vi "S4GUI.vi"(7 "Tab ObsEng":enum32{"Obs", "CCD modes", "Eng"}(tab)) -> ()   [LabVIEW 2018] (continued)
                    n784 = property on="Vertical Binning 2" class="DigNum (strict)"("Blinking"=w1441) -> ()  [unwired: 2 in, 2 out]
                    n785 = property on="Horizontal Binning 2" class="DigNum (strict)"("Blinking"=w1443) -> ()  [unwired: 2 in, 2 out]
                    n786 = property on="CCD EM Gain 2" class="DigNum (strict)"("Blinking"=w1438) -> ()  [unwired: 2 in, 2 out]
                    n787 = property on="Shutter Mode 2" class="Ring (strict)"("Blinking"=w1439) -> ()  [unwired: 2 in, 2 out]
                    n788 = property on="Shutter TTL 2" class="Ring (strict)"("Blinking"=w1437) -> ()  [unwired: 2 in, 2 out]
                    n789 = Not(x=w1415) -> (.not. x?=w1430:bool)
                    n790 = Not(x=w1411) -> (.not. x?=w1433:bool)
                    n791 = Not(x=w1410) -> (.not. x?=w1431:bool)
                    n792 = Not(x=w1409) -> (.not. x?=w1432:bool)
                    n793 = Not(x=w1414) -> (.not. x?=w1435:bool)
                    n794 = Not(x=w1413) -> (.not. x?=w1434:bool)
                    n795 = Not(x=w1412) -> (.not. x?=w1436:bool)
                    n796 = property on="Acquisition Mode 2" class="Ring (strict)"("Blinking"=w1430) -> ()  [unwired: 2 in, 2 out]
                    n797 = property on="Readout Rate 2" class="Ring (strict)"("Blinking"=w1433) -> ()  [unwired: 2 in, 2 out]
                    n798 = property on="Vertical Shift Speed 2" class="Ring (strict)"("Blinking"=w1431) -> ()  [unwired: 2 in, 2 out]
                    n799 = property on="CCD EM Mode 2" class="Ring (strict)"("Blinking"=w1432) -> ()  [unwired: 2 in, 2 out]
                    n800 = property on="Trigger Mode 2" class="Ring (strict)"("Blinking"=w1435) -> ()  [unwired: 2 in, 2 out]
                    n801 = property on="Read Mode 2" class="Ring (strict)"("Blinking"=w1434) -> ()  [unwired: 2 in, 2 out]
                    n802 = property on="Pre-amplification Gain 2" class="Ring (strict)"("Blinking"=w1436) -> ()  [unwired: 2 in, 2 out]
                  }
                }
                n803 = local read "Cameras Cluster"() -> (w1400:T7)
                n804 = Bundle By Name(cluster=w1400, "Current Configuration.Image Initial Line 2"=w1363, "Current Configuration.Image Initial Column 2"=w1361, "Current Configuration.Image Final Line 2"=w1364, "Current Configuration.Image FInal Column 2"=w1362, "Current Configuration.Vertical Binning 2"=w1367, "Current Configuration.Horizontal Binning 2"=w1398, "Current Configuration.Pre-amplification Gain 2"=w1366, "Current Configuration.CCD EM Gain 2"=w1365, "Current Configuration.Readout Rate 2"=w1360, "Current Configuration.Shutter Openning Time 2"=w1397, "Current Configuration.Shutter Closing Time 2"=w1396, "Current Configuration.Vertical Shift Speed 2"=w1395, "Current Configuration.Read Mode 2"=w1394, "Current Configuration.Vertical Clock Voltage 2"=w1393, "Current Configuration.A/D Channel 2"=w1392, "Current Configuration.Shutter Mode 2"=w1389, "Current Configuration.Shutter TTL 2"=w1390, "Current Configuration.Trigger Mode 2"=w1368, "Current Configuration.Frame Transfer 2"=w1369, "Current Configuration.Acquisition Mode 2"=w1391, "Current Configuration.CCD EM Mode 2"=w1359) -> (w1399:T7)
                n805 = local write "PA2"(w1354) -> ()
                n806 = local write "B2"(w1353) -> ()
                n807 = local write "EA2"(w1355) -> ()
                n808 = local write "SI2"(w1350) -> ()
                n809 = local write "RO2"(w1351) -> ()
                n810 = local write "G2"(w1352) -> ()
                n811 = local write "Cameras Cluster"(w1399) -> ()
                n812 = Compound Arithmetic op=AND(w1374, w1373, w1372, w1371, w1347, w1346, w1370, w1381, w1380, w1379, w1378, w1377, w1376, w1375, w1388, w1387, w1386, w1385, w1384, w1383, w1382) -> (w1345:bool)
                "CCD checked 2" <- w1345
                n813 = disable-structure shown="Disabled" {
                  disable-tunnel: w1345 -> [w1402 _]
                  frame Disabled {
                    n814 = Select(t=u32 1244955, s=w1402, f=u32 16718848) -> (s? t:f=w1405:u32)
                    n815 = property on="CCD checked 2" class="Bool (strict)"("Caption.BG Color"=w1405) -> ()  [unwired: 2 in, 2 out]
                  }
                  frame Enabled {
                  }
                }
                n816 = property on="Acquisition Mode 2" class="Ring (strict)"("DisabledEnum"=w1348) -> ()  [unwired: 2 in, 2 out]
                n817 = property on="Readout Rate 2" class="Ring (strict)"("DisabledEnum"=w1348) -> ()  [unwired: 2 in, 2 out]
                n818 = property on="Vertical Shift Speed 2" class="Ring (strict)"("DisabledEnum"=w1348) -> ()  [unwired: 2 in, 2 out]
                n819 = property on="CCD EM Mode 2" class="Ring (strict)"("DisabledEnum"=w1348) -> ()  [unwired: 2 in, 2 out]
                n820 = property on="Shutter Openning Time 2" class="DigNum (strict)"("DisabledEnum"=w1348) -> ()  [unwired: 2 in, 2 out]
                n821 = property on="Shutter Closing Time 2" class="DigNum (strict)"("DisabledEnum"=w1348) -> ()  [unwired: 2 in, 2 out]
                n822 = property on="Vertical Binning 2" class="DigNum (strict)"("DisabledEnum"=w1348) -> ()  [unwired: 2 in, 2 out]
                n823 = property on="Horizontal Binning 2" class="DigNum (strict)"("DisabledEnum"=w1348) -> ()  [unwired: 2 in, 2 out]
                n824 = property on="Trigger Mode 2" class="Ring (strict)"("DisabledEnum"=w1348) -> ()  [unwired: 2 in, 2 out]
                n825 = property on="Read Mode 2" class="Ring (strict)"("DisabledEnum"=w1348) -> ()  [unwired: 2 in, 2 out]
                n826 = property on="Pre-amplification Gain 2" class="Ring (strict)"("DisabledEnum"=w1348) -> ()  [unwired: 2 in, 2 out]
                n827 = property on="CCD EM Gain 2" class="DigNum (strict)"("DisabledEnum"=w1348) -> ()  [unwired: 2 in, 2 out]
                n828 = property on="Shutter Mode 2" class="Ring (strict)"("DisabledEnum"=w1348) -> ()  [unwired: 2 in, 2 out]
                n829 = property on="Shutter TTL 2" class="Ring (strict)"("DisabledEnum"=w1348) -> ()  [unwired: 2 in, 2 out]
                n830 = property on="Image FInal Column 2" class="DigNum (strict)"("DisabledEnum"=w1348) -> ()  [unwired: 2 in, 2 out]
                n831 = property on="Frame Transfer 2" class="Bool (strict)"("DisabledEnum"=w1348) -> ()  [unwired: 2 in, 2 out]
                n832 = property on="Vertical Clock Voltage 2" class="Ring (strict)"("DisabledEnum"=w1348) -> ()  [unwired: 2 in, 2 out]
                n833 = property on="A/D Channel 2" class="DigNum (strict)"("DisabledEnum"=w1348) -> ()  [unwired: 2 in, 2 out]
                n834 = property on="Image Initial Line 2" class="DigNum (strict)"("DisabledEnum"=w1348) -> ()  [unwired: 2 in, 2 out]
                n835 = property on="Image Initial Column 2" class="DigNum (strict)"("DisabledEnum"=w1348) -> ()  [unwired: 2 in, 2 out]
                n836 = property on="Image Final Line 2" class="DigNum (strict)"("DisabledEnum"=w1348) -> ()  [unwired: 2 in, 2 out]
              }
              frame #17 {
                # "Carrega coluna do Channel 3"
                # "Aba:  Eng->Camera"
                n837 = Unbundle By Name(w1564) -> ("ChannelC_CCD"=w1534:T28, "CHC_Checked Params"=w1549:T14, "ChannelC_Status.connection"=w1527:bool)
                n838 = Unbundle By Name(w1549) -> ("ACQUISITION_MODE"=w1516:bool, "TRIGGER_MODE"=w1515:bool, "READ_MODE"=w1514:bool, "PREAMP"=w1513:bool, "READOUT_RATE"=w1512:bool, "VERTICAL_SHIFT_SPEED"=w1511:bool, "EM_MODE"=w1510:bool, "EM_GAIN"=w1547:bool, "SHUTTER_MODE"=w1546:bool, "SHUTTER_TTL"=w1545:bool, "SHUTTER_OPENING_TIME"=w1544:bool, "SHUTTER_CLOSING_TIME"=w1526:bool, "VBIN"=w1518:bool, "HBIN"=w1517:bool, "INITIAL_LINE"=w1525:bool, "INITIAL_COLUMN"=w1524:bool, "FINAL_LINE"=w1523:bool, "FINAL_COLUMN"=w1522:bool, "FRAME_TRANSFER"=w1521:bool, "VERTICAL_CLOCK_VOLTAGE"=w1520:bool, "AD_CHANNEL"=w1519:bool)
                n839 = case shown="True" w1527 {
                  tunnel: w1534 -> [_ w1617]
                  tunnel: [w1610 w1616] -> w1533
                  tunnel: [w1610 w1615] -> w1532
                  tunnel: [w1610 w1614] -> w1531
                  tunnel: [w1610 w1613] -> w1530
                  tunnel: [w1610 w1612] -> w1529
                  tunnel: [w1610 w1611] -> w1528
                  frame False {
                    w1610 = ""
                  }
                  frame True {
                    n840 = stacked-sequence "Atualizacao dos indicadores inferiores do CANAL C da tela principal" {
                      tunnel: w1617 -> [w1632 w1635 w1640 w1649 w1652 w1656]
                      tunnel: [w1618 _ _ _ _ _] -> w1616
                      tunnel: [_ w1633 _ _ _ _] -> w1615
                      tunnel: [_ _ w1638 _ _ _] -> w1614
                      tunnel: [_ _ _ w1643 _ _] -> w1613
                      tunnel: [_ _ _ _ w1650 _] -> w1612
                      tunnel: [_ _ _ _ _ w1653] -> w1611
                      frame #0 {
                        # "SubImage"
                        n841 = Unbundle By Name(w1632) -> ("INITIAL_LINE"=w1630:u16, "FINAL_LINE"=w1629:u16, "INITIAL_COLUMN"=w1628:u16, "FINAL_COLUMN"=w1627:u16)
                        n842 = Number To Decimal String(number=w1630) -> (decimal integer string=w1626:string)  [unwired: 1 in]
                        n843 = Number To Decimal String(number=w1629) -> (decimal integer string=w1624:string)  [unwired: 1 in]
                        n844 = Number To Decimal String(number=w1628) -> (decimal integer string=w1622:string)  [unwired: 1 in]
                        n845 = Number To Decimal String(number=w1627) -> (decimal integer string=w1620:string)  [unwired: 1 in]
                        n846 = Concatenate Strings("[", w1626, ":", w1624, ",", w1622, ":", w1620, "]") -> (w1618:string)
                      }
                      frame #1 {
                        # "Em Active"
                        n847 = Unbundle By Name(w1635) -> ("EM_MODE"=w1634:u8)
                        n848 = case shown="0, Default" w1634 {
                          tunnel: ["Electron M." ("EmActive1") "Convent." ("EmActive1")] -> w1633
                          frame 0, Default {
                          }
                          frame 1 {
                          }
                        }
                      }
                      frame #2 {
                        # "Pre Amp"
                        n849 = Unbundle By Name(w1640) -> ("PREAMP"=w1639:u8)
                        n850 = case shown="1" w1639 {
                          tunnel: ["Gain 1" ("EmActive1") "Gain 2" ("EmActive1")] -> w1638
                          frame 0, Default {
                          }
                          frame 1 {
                          }
                        }
                      }
                      frame #3 {
                        # "Binning"
                        n851 = Unbundle By Name(w1649) -> ("VBIN"=w1648:u16, "HBIN"=w1647:u16)
                        n852 = Number To Decimal String(number=w1647) -> (decimal integer string=w1644:string)  [unwired: 1 in]
                        n853 = Number To Decimal String(number=w1648) -> (decimal integer string=w1646:string)  [unwired: 1 in]
                        n854 = Concatenate Strings(w1646, "x", w1644) -> (w1643:string)
                      }
                      frame #4 {
                        # "Gain"
                        n855 = Unbundle By Name(w1652) -> ("EM_GAIN"=w1651:u16)
                        n856 = Number To Decimal String(number=w1651) -> (decimal integer string=w1650:string)  [unwired: 1 in]
                      }
                      frame #5 {
                        # "Readout"
                        n857 = Unbundle By Name(w1656) -> ("EM_MODE"=w1655:u8, "READOUT_RATE"=w1654:u8)
                        n858 = case shown="0, Default" w1655 {
                          tunnel: w1654 -> [w1658 w1664]
                          tunnel: [w1657 w1663] -> w1653
                          frame 0, Default {
                            n859 = case shown="3" w1658 {
                              tunnel: ["30 MHz" ("EmActive1") "20 MHz" ("EmActive1") "10 MHz" ("EmActive1") "1 MHz" ("EmActive1")] -> w1657
                              frame 0, Default {
                              }
                              frame 1 {
                              }
                              frame 2 {
                              }
                              frame 3 {
                              }
                            }
                          }
                          frame 1 {
                            n860 = case shown="1" w1664 {
                              tunnel: ["1 MHz" ("EmActive1") "0.1 MHz" ("EmActive1")] -> w1663
                              frame 0, Default {
                              }
                              frame 1 {
                              }
                            }
                          }
                        }
                      }
                    }
                  }
                }
                n861 = Unbundle By Name(w1534) -> ("INITIAL_LINE"=w1539:u16, "INITIAL_COLUMN"=w1537:u16, "FINAL_LINE"=w1540:u16, "FINAL_COLUMN"=w1538:u16, "VBIN"=w1543:u16, "HBIN"=w1561:u16, "PREAMP"=w1542:u8, "EM_GAIN"=w1541:u16, "READOUT_RATE"=w1536:u8, "SHUTTER_OPENNING_TIME"=w1560:u16, "SHUTTER_CLOSING_TIME"=w1559:u16, "VERTICAL_SHIFT_SPEED"=w1558:u8, "READ_MODE"=w1557:u8, "VERTICAL_CLOCK_VOLTAGE"=w1556:u8, "AD_CHANNEL"=w1555:u32, "SHUTTER_MODE"=w1550:u8, "SHUTTER_TTL"=w1551:u8, "TRIGGER_MODE"=w1552:u8, "FRAME_TRANSFER"=w1553:bool, "ACQUISITION_MODE"=w1554:u8, "EM_MODE"=w1535:u8)
                n862 = local read "CH3 on"() -> (w1509:bool)
                n863 = case shown="True" w1509 {
                  tunnel: w1547 -> [_ w1590]
                  tunnel: w1546 -> [_ w1589]
                  tunnel: w1545 -> [_ w1587]
                  tunnel: w1544 -> [_ w1586]
                  tunnel: w1526 -> [_ w1585]
                  tunnel: w1525 -> [_ w1584]
                  tunnel: w1524 -> [_ w1583]
                  tunnel: w1523 -> [_ w1582]
                  tunnel: w1522 -> [_ w1581]
                  tunnel: w1521 -> [_ w1580]
                  tunnel: w1520 -> [_ w1579]
                  tunnel: w1519 -> [_ w1578]
                  tunnel: w1518 -> [_ w1577]
                  tunnel: w1517 -> [_ w1576]
                  tunnel: w1516 -> [_ w1575]
                  tunnel: w1515 -> [_ w1574]
                  tunnel: w1514 -> [_ w1573]
                  tunnel: w1513 -> [_ w1572]
                  tunnel: w1512 -> [_ w1571]
                  tunnel: w1511 -> [_ w1570]
                  tunnel: w1510 -> [_ w1569]
                  tunnel: [T12."Disabled and Grayed Out" ("Disabled") T12."Enabled" ("Disabled")] -> w1508
                  frame False {
                    w1565 = FALSE
                    n864 = property on="Image Initial Line 3" class="DigNum (strict)"("Blinking"=w1565) -> ()  [unwired: 2 in, 2 out]
                    n865 = property on="Image Initial Column 3" class="DigNum (strict)"("Blinking"=w1565) -> ()  [unwired: 2 in, 2 out]
                    n866 = property on="Image Final Line 3" class="DigNum (strict)"("Blinking"=w1565) -> ()  [unwired: 2 in, 2 out]
                    n867 = property on="Image FInal Column 3" class="DigNum (strict)"("Blinking"=w1565) -> ()  [unwired: 2 in, 2 out]
                    n868 = property on="Frame Transfer 3" class="Bool (strict)"("Blinking"=w1565) -> ()  [unwired: 2 in, 2 out]
                    n869 = property on="Vertical Clock Voltage 3" class="Ring (strict)"("Blinking"=w1565) -> ()  [unwired: 2 in, 2 out]
                    n870 = property on="A/D Channel 3" class="DigNum (strict)"("Blinking"=w1565) -> ()  [unwired: 2 in, 2 out]
                    n871 = property on="CCD EM Gain 3" class="DigNum (strict)"("Blinking"=w1565) -> ()  [unwired: 2 in, 2 out]
                    n872 = property on="Shutter Mode 3" class="Ring (strict)"("Blinking"=w1565) -> ()  [unwired: 2 in, 2 out]
                    n873 = property on="Shutter TTL 3" class="Ring (strict)"("Blinking"=w1565) -> ()  [unwired: 2 in, 2 out]
                    n874 = property on="Shutter Openning Time 3" class="DigNum (strict)"("Blinking"=w1565) -> ()  [unwired: 2 in, 2 out]
                    n875 = property on="Shutter Closing Time 3" class="DigNum (strict)"("Blinking"=w1565) -> ()  [unwired: 2 in, 2 out]
                    n876 = property on="Vertical Binning 3" class="DigNum (strict)"("Blinking"=w1565) -> ()  [unwired: 2 in, 2 out]
                    n877 = property on="Horizontal Binning 3" class="DigNum (strict)"("Blinking"=w1565) -> ()  [unwired: 2 in, 2 out]
                    n878 = property on="Acquisition Mode 3" class="Ring (strict)"("Blinking"=w1565) -> ()  [unwired: 2 in, 2 out]
                    n879 = property on="Vertical Shift Speed 3" class="Ring (strict)"("Blinking"=w1565) -> ()  [unwired: 2 in, 2 out]
                    n880 = property on="Trigger Mode 3" class="Ring (strict)"("Blinking"=w1565) -> ()  [unwired: 2 in, 2 out]
                    n881 = property on="Read Mode 3" class="Ring (strict)"("Blinking"=w1565) -> ()  [unwired: 2 in, 2 out]
                    n882 = property on="Readout Rate 3" class="Ring (strict)"("Blinking"=w1565) -> ()  [unwired: 2 in, 2 out]
                    n883 = property on="CCD EM Mode 3" class="Ring (strict)"("Blinking"=w1565) -> ()  [unwired: 2 in, 2 out]
                    n884 = property on="Pre-amplification Gain 3" class="Ring (strict)"("Blinking"=w1565) -> ()  [unwired: 2 in, 2 out]
                  }
                  frame True {
                    n885 = Not(x=w1584) -> (.not. x?=w1567:bool)
                    n886 = Not(x=w1583) -> (.not. x?=w1608:bool)
                    n887 = Not(x=w1582) -> (.not. x?=w1609:bool)
                    n888 = Not(x=w1581) -> (.not. x?=w1607:bool)
                    n889 = Not(x=w1580) -> (.not. x?=w1605:bool)
                    n890 = Not(x=w1579) -> (.not. x?=w1606:bool)
                    n891 = Not(x=w1578) -> (.not. x?=w1604:bool)
                    n892 = property on="Image FInal Column 3" class="DigNum (strict)"("Blinking"=w1607) -> ()  [unwired: 2 in, 2 out]
                    n893 = property on="Frame Transfer 3" class="Bool (strict)"("Blinking"=w1605) -> ()  [unwired: 2 in, 2 out]
                    n894 = property on="Vertical Clock Voltage 3" class="Ring (strict)"("Blinking"=w1606) -> ()  [unwired: 2 in, 2 out]
                    n895 = property on="Image Initial Line 3" class="DigNum (strict)"("Blinking"=w1567) -> ()  [unwired: 2 in, 2 out]
                    n896 = property on="Image Initial Column 3" class="DigNum (strict)"("Blinking"=w1608) -> ()  [unwired: 2 in, 2 out]
                    n897 = property on="Image Final Line 3" class="DigNum (strict)"("Blinking"=w1609) -> ()  [unwired: 2 in, 2 out]
                    n898 = property on="A/D Channel 3" class="DigNum (strict)"("Blinking"=w1604) -> ()  [unwired: 2 in, 2 out]
                    n899 = Not(x=w1586) -> (.not. x?=w1600:bool)
                    n900 = Not(x=w1585) -> (.not. x?=w1602:bool)
                    n901 = Not(x=w1577) -> (.not. x?=w1601:bool)
                    n902 = Not(x=w1576) -> (.not. x?=w1603:bool)
                    n903 = Not(x=w1590) -> (.not. x?=w1599:bool)
                    n904 = Not(x=w1589) -> (.not. x?=w1588:bool)
                    n905 = Not(x=w1587) -> (.not. x?=w1598:bool)
                    n906 = property on="Shutter Openning Time 3" class="DigNum (strict)"("Blinking"=w1600) -> ()  [unwired: 2 in, 2 out]
                    n907 = property on="Shutter Closing Time 3" class="DigNum (strict)"("Blinking"=w1602) -> ()  [unwired: 2 in, 2 out]
                    n908 = property on="Vertical Binning 3" class="DigNum (strict)"("Blinking"=w1601) -> ()  [unwired: 2 in, 2 out]
                    n909 = property on="Horizontal Binning 3" class="DigNum (strict)"("Blinking"=w1603) -> ()  [unwired: 2 in, 2 out]
                    n910 = property on="CCD EM Gain 3" class="DigNum (strict)"("Blinking"=w1599) -> ()  [unwired: 2 in, 2 out]
                    n911 = property on="Shutter Mode 3" class="Ring (strict)"("Blinking"=w1588) -> ()  [unwired: 2 in, 2 out]
                    n912 = property on="Shutter TTL 3" class="Ring (strict)"("Blinking"=w1598) -> ()  [unwired: 2 in, 2 out]
                    n913 = Not(x=w1575) -> (.not. x?=w1591:bool)
                    n914 = Not(x=w1571) -> (.not. x?=w1594:bool)
                    n915 = Not(x=w1570) -> (.not. x?=w1592:bool)
                    n916 = Not(x=w1569) -> (.not. x?=w1593:bool)
                    n917 = Not(x=w1574) -> (.not. x?=w1596:bool)
                    n918 = Not(x=w1573) -> (.not. x?=w1595:bool)
                    n919 = Not(x=w1572) -> (.not. x?=w1597:bool)
                    n920 = property on="Acquisition Mode 3" class="Ring (strict)"("Blinking"=w1591) -> ()  [unwired: 2 in, 2 out]
                    n921 = property on="Readout Rate 3" class="Ring (strict)"("Blinking"=w1594) -> ()  [unwired: 2 in, 2 out]
                    n922 = property on="Vertical Shift Speed 3" class="Ring (strict)"("Blinking"=w1592) -> ()  [unwired: 2 in, 2 out]
                    n923 = property on="CCD EM Mode 3" class="Ring (strict)"("Blinking"=w1593) -> ()  [unwired: 2 in, 2 out]
                    n924 = property on="Trigger Mode 3" class="Ring (strict)"("Blinking"=w1596) -> ()  [unwired: 2 in, 2 out]
                    n925 = property on="Read Mode 3" class="Ring (strict)"("Blinking"=w1595) -> ()  [unwired: 2 in, 2 out]
                    n926 = property on="Pre-amplification Gain 3" class="Ring (strict)"("Blinking"=w1597) -> ()  [unwired: 2 in, 2 out]
                  }
                }
                n927 = local write "RO3"(w1528) -> ()
                n928 = local write "B3"(w1530) -> ()
                n929 = local write "PA3"(w1531) -> ()
                n930 = local write "EA3"(w1532) -> ()
                n931 = local write "G3"(w1529) -> ()
                n932 = local write "SI3"(w1533) -> ()
                n933 = local read "Cameras Cluster"() -> (w1563:T7)
                n934 = Bundle By Name(cluster=w1563, "Current Configuration.Image Initial Line 3"=w1539, "Current Configuration.Image Initial Column 3"=w1537, "Current Configuration.Image Final Line 3"=w1540, "Current Configuration.Image FInal Column 3"=w1538, "Current Configuration.Vertical Binning 3"=w1543, "Current Configuration.Horizontal Binning 3"=w1561, "Current Configuration.Pre-amplification Gain 3"=w1542, "Current Configuration.CCD EM Gain 3"=w1541, "Current Configuration.Readout Rate 3"=w1536, "Current Configuration.Shutter Openning Time 3"=w1560, "Current Configuration.Shutter Closing Time 3"=w1559, "Current Configuration.Vertical Shift Speed 3"=w1558, "Current Configuration.Read Mode 3"=w1557, "Current Configuration.Vertical Clock Voltage 3"=w1556, "Current Configuration.A/D Channel 3"=w1555, "Current Configuration.Shutter Mode 3"=w1550, "Current Configuration.Shutter TTL 3"=w1551, "Current Configuration.Trigger Mode 3"=w1552, "Current Configuration.Frame Transfer 3"=w1553, "Current Configuration.Acquisition Mode 3"=w1554, "Current Configuration.CCD EM Mode 3"=w1535) -> (w1562:T7)
                n935 = local write "Cameras Cluster"(w1562) -> ()
                n936 = Compound Arithmetic op=AND(w1516, w1515, w1514, w1513, w1512, w1511, w1510, w1547, w1546, w1545, w1544, w1526, w1518, w1517, w1525, w1524, w1523, w1522, w1521, w1520, w1519) -> (→"CCD checked 3":bool)
                n937 = property on="Image Initial Line 3" class="DigNum (strict)"("DisabledEnum"=w1508) -> ()  [unwired: 2 in, 2 out]
                n938 = property on="Image Initial Column 3" class="DigNum (strict)"("DisabledEnum"=w1508) -> ()  [unwired: 2 in, 2 out]
                n939 = property on="Image Final Line 3" class="DigNum (strict)"("DisabledEnum"=w1508) -> ()  [unwired: 2 in, 2 out]
                n940 = property on="Image FInal Column 3" class="DigNum (strict)"("DisabledEnum"=w1508) -> ()  [unwired: 2 in, 2 out]
                n941 = property on="Frame Transfer 3" class="Bool (strict)"("DisabledEnum"=w1508) -> ()  [unwired: 2 in, 2 out]
                n942 = property on="Horizontal Binning 3" class="DigNum (strict)"("DisabledEnum"=w1508) -> ()  [unwired: 2 in, 2 out]
                n943 = property on="Vertical Clock Voltage 3" class="Ring (strict)"("DisabledEnum"=w1508) -> ()  [unwired: 2 in, 2 out]
                n944 = property on="CCD EM Gain 3" class="DigNum (strict)"("DisabledEnum"=w1508) -> ()  [unwired: 2 in, 2 out]
                n945 = property on="Shutter Mode 3" class="Ring (strict)"("DisabledEnum"=w1508) -> ()  [unwired: 2 in, 2 out]
                n946 = property on="Shutter Openning Time 3" class="DigNum (strict)"("DisabledEnum"=w1508) -> ()  [unwired: 2 in, 2 out]
                n947 = property on="Shutter Closing Time 3" class="DigNum (strict)"("DisabledEnum"=w1508) -> ()  [unwired: 2 in, 2 out]
                n948 = property on="Vertical Binning 3" class="DigNum (strict)"("DisabledEnum"=w1508) -> ()  [unwired: 2 in, 2 out]
                n949 = property on="Shutter TTL 3" class="Ring (strict)"("DisabledEnum"=w1508) -> ()  [unwired: 2 in, 2 out]
                n950 = property on="Pre-amplification Gain 3" class="Ring (strict)"("DisabledEnum"=w1508) -> ()  [unwired: 2 in, 2 out]
                n951 = property on="Acquisition Mode 3" class="Ring (strict)"("DisabledEnum"=w1508) -> ()  [unwired: 2 in, 2 out]
                n952 = property on="Trigger Mode 3" class="Ring (strict)"("DisabledEnum"=w1508) -> ()  [unwired: 2 in, 2 out]
                n953 = property on="Read Mode 3" class="Ring (strict)"("DisabledEnum"=w1508) -> ()  [unwired: 2 in, 2 out]
                n954 = property on="Readout Rate 3" class="Ring (strict)"("DisabledEnum"=w1508) -> ()  [unwired: 2 in, 2 out]
                n955 = property on="A/D Channel 3" class="DigNum (strict)"("DisabledEnum"=w1508) -> ()  [unwired: 2 in, 2 out]
                n956 = property on="Vertical Shift Speed 3" class="Ring (strict)"("DisabledEnum"=w1508) -> ()  [unwired: 2 in, 2 out]
                n957 = property on="CCD EM Mode 3" class="Ring (strict)"("DisabledEnum"=w1508) -> ()  [unwired: 2 in, 2 out]
              }
              frame #18 {
                # "Carrega coluna do Channel 4"
                # "Aba:  Eng->Camera"
                n958 = Unbundle By Name(w1723) -> ("ChannelD_CCD"=w1676:T28, "CHD_Checked Params"=w1708:T14, "ChannelD_Status.connection"=w1675:bool)
                n959 = Unbundle By Name(w1708) -> ("ACQUISITION_MODE"=w1692:bool, "TRIGGER_MODE"=w1691:bool, "READ_MODE"=w1690:bool, "PREAMP"=w1689:bool, "READOUT_RATE"=w1688:bool, "VERTICAL_SHIFT_SPEED"=w1687:bool, "EM_MODE"=w1686:bool, "EM_GAIN"=w1699:bool, "SHUTTER_MODE"=w1698:bool, "SHUTTER_TTL"=w1697:bool, "SHUTTER_OPENING_TIME"=w1696:bool, "SHUTTER_CLOSING_TIME"=w1695:bool, "VBIN"=w1694:bool, "HBIN"=w1693:bool, "INITIAL_LINE"=w1706:bool, "INITIAL_COLUMN"=w1705:bool, "FINAL_LINE"=w1704:bool, "FINAL_COLUMN"=w1703:bool, "FRAME_TRANSFER"=w1702:bool, "VERTICAL_CLOCK_VOLTAGE"=w1701:bool, "AD_CHANNEL"=w1700:bool)
                n960 = case shown="True" w1675 {
                  tunnel: w1676 -> [_ w1776]
                  tunnel: [w1769 w1775] -> w1674
                  tunnel: [w1769 w1774] -> w1673
                  tunnel: [w1769 w1773] -> w1672
                  tunnel: [w1769 w1772] -> w1671
                  tunnel: [w1769 w1771] -> w1670
                  tunnel: [w1769 w1770] -> w1669
                  frame False {
                    w1769 = ""
                  }
                  frame True {
                    n961 = stacked-sequence "Atualizacao dos indicadores inferiores do CANAL D da tela principal" {
                      tunnel: w1776 -> [w1791 w1794 w1799 w1808 w1811 w1815]
                      tunnel: [w1777 _ _ _ _ _] -> w1775
                      tunnel: [_ w1792 _ _ _ _] -> w1774
                      tunnel: [_ _ w1797 _ _ _] -> w1773
                      tunnel: [_ _ _ w1802 _ _] -> w1772
                      tunnel: [_ _ _ _ w1809 _] -> w1771
                      tunnel: [_ _ _ _ _ w1812] -> w1770
                      frame #0 {
                        # "SubImage"
                        n962 = Unbundle By Name(w1791) -> ("INITIAL_LINE"=w1789:u16, "FINAL_LINE"=w1788:u16, "INITIAL_COLUMN"=w1787:u16, "FINAL_COLUMN"=w1786:u16)
                        n963 = Number To Decimal String(number=w1789) -> (decimal integer string=w1785:string)  [unwired: 1 in]
                        n964 = Number To Decimal String(number=w1788) -> (decimal integer string=w1783:string)  [unwired: 1 in]
                        n965 = Number To Decimal String(number=w1787) -> (decimal integer string=w1781:string)  [unwired: 1 in]
                        n966 = Number To Decimal String(number=w1786) -> (decimal integer string=w1779:string)  [unwired: 1 in]
                        n967 = Concatenate Strings("[", w1785, ":", w1783, ",", w1781, ":", w1779, "]") -> (w1777:string)
                      }
                      frame #1 {
                        # "Em Active"
                        n968 = Unbundle By Name(w1794) -> ("EM_MODE"=w1793:u8)
                        n969 = case shown="0, Default" w1793 {
                          tunnel: ["Electron M." ("EmActive1") "Convent." ("EmActive1")] -> w1792
                          frame 0, Default {
                          }
                          frame 1 {
                          }
                        }
                      }
                      frame #2 {
                        # "Pre Amp"
                        n970 = Unbundle By Name(w1799) -> ("PREAMP"=w1798:u8)
                        n971 = case shown="1" w1798 {
                          tunnel: ["Gain 1" ("EmActive1") "Gain 2" ("EmActive1")] -> w1797
                          frame 0, Default {
                          }
                          frame 1 {
                          }
                        }
                      }
                      frame #3 {
                        # "Binning"
                        n972 = Unbundle By Name(w1808) -> ("VBIN"=w1807:u16, "HBIN"=w1806:u16)
                        n973 = Number To Decimal String(number=w1806) -> (decimal integer string=w1803:string)  [unwired: 1 in]
                        n974 = Number To Decimal String(number=w1807) -> (decimal integer string=w1805:string)  [unwired: 1 in]
                        n975 = Concatenate Strings(w1805, "x", w1803) -> (w1802:string)
                      }
                      frame #4 {
                        # "Gain"
                        n976 = Unbundle By Name(w1811) -> ("EM_GAIN"=w1810:u16)
                        n977 = Number To Decimal String(number=w1810) -> (decimal integer string=w1809:string)  [unwired: 1 in]
                      }
                      frame #5 {
                        # "Readout"
                        n978 = Unbundle By Name(w1815) -> ("EM_MODE"=w1814:u8, "READOUT_RATE"=w1813:u8)
                        n979 = case shown="0, Default" w1814 {
                          tunnel: w1813 -> [w1817 w1823]
                          tunnel: [w1816 w1822] -> w1812
                          frame 0, Default {
                            n980 = case shown="3" w1817 {
                              tunnel: ["30 MHz" ("EmActive1") "20 MHz" ("EmActive1") "10 MHz" ("EmActive1") "1 MHz" ("EmActive1")] -> w1816
                              frame 0, Default {
                              }
                              frame 1 {
                              }
                              frame 2 {
                              }
                              frame 3 {
                              }
                            }
                          }
                          frame 1 {
                            n981 = case shown="0, Default" w1823 {
                              tunnel: ["1 MHz" ("EmActive1") "0.1 MHz" ("EmActive1")] -> w1822
                              frame 0, Default {
                              }
                              frame 1 {
                              }
                            }
                          }
                        }
                      }
                    }
                  }
                }
                n982 = Unbundle By Name(w1676) -> ("INITIAL_LINE"=w1681:u16, "INITIAL_COLUMN"=w1679:u16, "FINAL_LINE"=w1682:u16, "FINAL_COLUMN"=w1680:u16, "VBIN"=w1685:u16, "HBIN"=w1720:u16, "PREAMP"=w1684:u8, "EM_GAIN"=w1683:u16, "READOUT_RATE"=w1678:u8, "SHUTTER_OPENNING_TIME"=w1719:u16, "SHUTTER_CLOSING_TIME"=w1718:u16, "VERTICAL_SHIFT_SPEED"=w1717:u8, "READ_MODE"=w1716:u8, "VERTICAL_CLOCK_VOLTAGE"=w1715:u8, "AD_CHANNEL"=w1714:u32, "SHUTTER_MODE"=w1709:u8, "SHUTTER_TTL"=w1710:u8, "TRIGGER_MODE"=w1711:u8, "FRAME_TRANSFER"=w1712:bool, "ACQUISITION_MODE"=w1713:u8, "EM_MODE"=w1677:u8)
                n983 = local read "CH4 on"() -> (w1668:bool)
                n984 = case shown="False" w1668 {
                  tunnel: w1706 -> [_ w1748]
                  tunnel: w1705 -> [_ w1747]
                  tunnel: w1704 -> [_ w1746]
                  tunnel: w1703 -> [_ w1745]
                  tunnel: w1702 -> [_ w1744]
                  tunnel: w1701 -> [_ w1743]
                  tunnel: w1700 -> [_ w1742]
                  tunnel: w1699 -> [_ w1741]
                  tunnel: w1698 -> [_ w1740]
                  tunnel: w1697 -> [_ w1739]
                  tunnel: w1696 -> [_ w1738]
                  tunnel: w1695 -> [_ w1737]
                  tunnel: w1694 -> [_ w1736]
                  tunnel: w1693 -> [_ w1735]
                  tunnel: w1692 -> [_ w1734]
                  tunnel: w1691 -> [_ w1733]
                  tunnel: w1690 -> [_ w1732]
                  tunnel: w1689 -> [_ w1730]
                  tunnel: w1688 -> [_ w1729]
                  tunnel: w1687 -> [_ w1728]
                  tunnel: w1686 -> [_ w1727]
                  tunnel: [T12."Disabled and Grayed Out" ("Disabled") T12."Enabled" ("Disabled")] -> w1667
                  frame False {
                    w1725 = FALSE ("Blinking")
                    n985 = property on="Image FInal Column 4" class="DigNum (strict)"("Blinking"=w1725) -> ()  [unwired: 2 in, 2 out]
                    n986 = property on="Frame Transfer 4" class="Bool (strict)"("Blinking"=w1725) -> ()  [unwired: 2 in, 2 out]
                    n987 = property on="Vertical Clock Voltage 4" class="Ring (strict)"("Blinking"=w1725) -> ()  [unwired: 2 in, 2 out]
                    n988 = property on="A/D Channel 4" class="DigNum (strict)"("Blinking"=w1725) -> ()  [unwired: 2 in, 2 out]
                    n989 = property on="Image Initial Line 4" class="DigNum (strict)"("Blinking"=w1725) -> ()  [unwired: 2 in, 2 out]
                    n990 = property on="Image Initial Column 4" class="DigNum (strict)"("Blinking"=w1725) -> ()  [unwired: 2 in, 2 out]
                    n991 = property on="Image Final Line 4" class="DigNum (strict)"("Blinking"=w1725) -> ()  [unwired: 2 in, 2 out]
                    n992 = property on="Shutter Openning Time 4" class="DigNum (strict)"("Blinking"=w1725) -> ()  [unwired: 2 in, 2 out]
                    n993 = property on="Shutter Closing Time 4" class="DigNum (strict)"("Blinking"=w1725) -> ()  [unwired: 2 in, 2 out]
                    n994 = property on="Vertical Binning 4" class="DigNum (strict)"("Blinking"=w1725) -> ()  [unwired: 2 in, 2 out]
                    n995 = property on="Horizontal Binning 4" class="DigNum (strict)"("Blinking"=w1725) -> ()  [unwired: 2 in, 2 out]
                    n996 = property on="CCD EM Gain 4" class="DigNum (strict)"("Blinking"=w1725) -> ()  [unwired: 2 in, 2 out]
                    n997 = property on="Shutter Mode 4" class="Ring (strict)"("Blinking"=w1725) -> ()  [unwired: 2 in, 2 out]
                    n998 = property on="Shutter TTL 4" class="Ring (strict)"("Blinking"=w1725) -> ()  [unwired: 2 in, 2 out]
                    n999 = property on="Acquisition Mode 4" class="Ring (strict)"("Blinking"=w1725) -> ()  [unwired: 2 in, 2 out]
                    n1000 = property on="Readout Rate 4" class="Ring (strict)"("Blinking"=w1725) -> ()  [unwired: 2 in, 2 out]
                    n1001 = property on="Vertical Shift Speed 4" class="Ring (strict)"("Blinking"=w1725) -> ()  [unwired: 2 in, 2 out]
                    n1002 = property on="CCD EM Mode 4" class="Ring (strict)"("Blinking"=w1725) -> ()  [unwired: 2 in, 2 out]
                    n1003 = property on="Trigger Mode 4" class="Ring (strict)"("Blinking"=w1725) -> ()  [unwired: 2 in, 2 out]
                    n1004 = property on="Read Mode 4" class="Ring (strict)"("Blinking"=w1725) -> ()  [unwired: 2 in, 2 out]
                    n1005 = property on="Pre-amplification Gain 4" class="Ring (strict)"("Blinking"=w1725) -> ()  [unwired: 2 in, 2 out]
                  }
                  frame True {
                    n1006 = Not(x=w1745) -> (.not. x?=w1765:bool)
                    n1007 = Not(x=w1744) -> (.not. x?=w1763:bool)
                    n1008 = Not(x=w1743) -> (.not. x?=w1764:bool)
                    n1009 = Not(x=w1742) -> (.not. x?=w1762:bool)
                    n1010 = Not(x=w1748) -> (.not. x?=w1767:bool)
                    n1011 = Not(x=w1747) -> (.not. x?=w1766:bool)
                    n1012 = Not(x=w1746) -> (.not. x?=w1768:bool)
                    n1013 = property on="Image FInal Column 4" class="DigNum (strict)"("Blinking"=w1765) -> ()  [unwired: 2 in, 2 out]
                    n1014 = property on="Frame Transfer 4" class="Bool (strict)"("Blinking"=w1763) -> ()  [unwired: 2 in, 2 out]
                    n1015 = property on="Vertical Clock Voltage 4" class="Ring (strict)"("Blinking"=w1764) -> ()  [unwired: 2 in, 2 out]
                    n1016 = property on="A/D Channel 4" class="DigNum (strict)"("Blinking"=w1762) -> ()  [unwired: 2 in, 2 out]
                    n1017 = property on="Image Initial Line 4" class="DigNum (strict)"("Blinking"=w1767) -> ()  [unwired: 2 in, 2 out]
                    n1018 = property on="Image Initial Column 4" class="DigNum (strict)"("Blinking"=w1766) -> ()  [unwired: 2 in, 2 out]
                    n1019 = property on="Image Final Line 4" class="DigNum (strict)"("Blinking"=w1768) -> ()  [unwired: 2 in, 2 out]
                    n1020 = Not(x=w1738) -> (.not. x?=w1758:bool)
                    n1021 = Not(x=w1737) -> (.not. x?=w1760:bool)
                    n1022 = Not(x=w1736) -> (.not. x?=w1759:bool)
                    n1023 = Not(x=w1735) -> (.not. x?=w1761:bool)
                    n1024 = Not(x=w1741) -> (.not. x?=w1756:bool)
                    n1025 = Not(x=w1740) -> (.not. x?=w1757:bool)
                    n1026 = Not(x=w1739) -> (.not. x?=w1755:bool)
                    n1027 = property on="Shutter Openning Time 4" class="DigNum (strict)"("Blinking"=w1758) -> ()  [unwired: 2 in, 2 out]
                    n1028 = property on="Shutter Closing Time 4" class="DigNum (strict)"("Blinking"=w1760) -> ()  [unwired: 2 in, 2 out]
                    n1029 = property on="Vertical Binning 4" class="DigNum (strict)"("Blinking"=w1759) -> ()  [unwired: 2 in, 2 out]
                    n1030 = property on="Horizontal Binning 4" class="DigNum (strict)"("Blinking"=w1761) -> ()  [unwired: 2 in, 2 out]
                    n1031 = property on="CCD EM Gain 4" class="DigNum (strict)"("Blinking"=w1756) -> ()  [unwired: 2 in, 2 out]
                    n1032 = property on="Shutter Mode 4" class="Ring (strict)"("Blinking"=w1757) -> ()  [unwired: 2 in, 2 out]
                    n1033 = property on="Shutter TTL 4" class="Ring (strict)"("Blinking"=w1755) -> ()  [unwired: 2 in, 2 out]
                    n1034 = Not(x=w1734) -> (.not. x?=w1749:bool)
                    n1035 = Not(x=w1729) -> (.not. x?=w1752:bool)
                    n1036 = Not(x=w1728) -> (.not. x?=w1750:bool)
                    n1037 = Not(x=w1727) -> (.not. x?=w1751:bool)
                    n1038 = Not(x=w1733) -> (.not. x?=w1753:bool)
                    n1039 = Not(x=w1732) -> (.not. x?=w1731:bool)
                    n1040 = Not(x=w1730) -> (.not. x?=w1754:bool)
                    n1041 = property on="Acquisition Mode 4" class="Ring (strict)"("Blinking"=w1749) -> ()  [unwired: 2 in, 2 out]
                    n1042 = property on="Readout Rate 4" class="Ring (strict)"("Blinking"=w1752) -> ()  [unwired: 2 in, 2 out]
                    n1043 = property on="Vertical Shift Speed 4" class="Ring (strict)"("Blinking"=w1750) -> ()  [unwired: 2 in, 2 out]
                    n1044 = property on="CCD EM Mode 4" class="Ring (strict)"("Blinking"=w1751) -> ()  [unwired: 2 in, 2 out]
                    n1045 = property on="Trigger Mode 4" class="Ring (strict)"("Blinking"=w1753) -> ()  [unwired: 2 in, 2 out]
                    n1046 = property on="Read Mode 4" class="Ring (strict)"("Blinking"=w1731) -> ()  [unwired: 2 in, 2 out]
                    n1047 = property on="Pre-amplification Gain 4" class="Ring (strict)"("Blinking"=w1754) -> ()  [unwired: 2 in, 2 out]
                  }
                }
                n1048 = local write "SI4"(w1674) -> ()
                n1049 = local write "RO4"(w1669) -> ()
                n1050 = local write "PA4"(w1672) -> ()
                n1051 = local write "EA4"(w1673) -> ()
                n1052 = local write "G4"(w1670) -> ()
                n1053 = local write "B4"(w1671) -> ()
                n1054 = local read "Cameras Cluster"() -> (w1722:T7)
                n1055 = Bundle By Name(cluster=w1722, "Current Configuration.Image Initial Line 4"=w1681, "Current Configuration.Image Initial Column 4"=w1679, "Current Configuration.Image Final Line 4"=w1682, "Current Configuration.Image FInal Column 4"=w1680, "Current Configuration.Vertical Binning 4"=w1685, "Current Configuration.Horizontal Binning 4"=w1720, "Current Configuration.Pre-amplification Gain 4"=w1684, "Current Configuration.CCD EM Gain 4"=w1683, "Current Configuration.Readout Rate 4"=w1678, "Current Configuration.Shutter Openning Time 4"=w1719, "Current Configuration.Shutter Closing Time 4"=w1718, "Current Configuration.Vertical Shift Speed 4"=w1717, "Current Configuration.Read Mode 4"=w1716, "Current Configuration.Vertical Clock Voltage 4"=w1715, "Current Configuration.A/D Channel 4"=w1714, "Current Configuration.Shutter Mode 4"=w1709, "Current Configuration.Shutter TTL 4"=w1710, "Current Configuration.Trigger Mode 4"=w1711, "Current Configuration.Frame Transfer 4"=w1712, "Current Configuration.Acquisition Mode 4"=w1713, "Current Configuration.CCD EM Mode 4"=w1677) -> (w1721:T7)
                n1056 = local write "Cameras Cluster"(w1721) -> ()
                n1057 = Compound Arithmetic op=AND(w1692, w1691, w1690, w1689, w1688, w1687, w1686, w1699, w1698, w1697, w1696, w1695, w1694, w1693, w1706, w1705, w1704, w1703, w1702, w1701, w1700) -> (→"CCD checked 4":bool)
                n1058 = property on="Image FInal Column 4" class="DigNum (strict)"("DisabledEnum"=w1667) -> ()  [unwired: 2 in, 2 out]
                n1059 = property on="Frame Transfer 4" class="Bool (strict)"("DisabledEnum"=w1667) -> ()  [unwired: 2 in, 2 out]
                n1060 = property on="Vertical Clock Voltage 4" class="Ring (strict)"("DisabledEnum"=w1667) -> ()  [unwired: 2 in, 2 out]
                n1061 = property on="A/D Channel 4" class="DigNum (strict)"("DisabledEnum"=w1667) -> ()  [unwired: 2 in, 2 out]
                n1062 = property on="Image Initial Line 4" class="DigNum (strict)"("DisabledEnum"=w1667) -> ()  [unwired: 2 in, 2 out]
                n1063 = property on="Image Initial Column 4" class="DigNum (strict)"("DisabledEnum"=w1667) -> ()  [unwired: 2 in, 2 out]
                n1064 = property on="Image Final Line 4" class="DigNum (strict)"("DisabledEnum"=w1667) -> ()  [unwired: 2 in, 2 out]
                n1065 = property on="Shutter Openning Time 4" class="DigNum (strict)"("DisabledEnum"=w1667) -> ()  [unwired: 2 in, 2 out]
                n1066 = property on="Shutter Closing Time 4" class="DigNum (strict)"("DisabledEnum"=w1667) -> ()  [unwired: 2 in, 2 out]
                n1067 = property on="Vertical Binning 4" class="DigNum (strict)"("DisabledEnum"=w1667) -> ()  [unwired: 2 in, 2 out]
                n1068 = property on="Horizontal Binning 4" class="DigNum (strict)"("DisabledEnum"=w1667) -> ()  [unwired: 2 in, 2 out]
                n1069 = property on="Acquisition Mode 4" class="Ring (strict)"("DisabledEnum"=w1667) -> ()  [unwired: 2 in, 2 out]
                n1070 = property on="CCD EM Gain 4" class="DigNum (strict)"("DisabledEnum"=w1667) -> ()  [unwired: 2 in, 2 out]
                n1071 = property on="Shutter Mode 4" class="Ring (strict)"("DisabledEnum"=w1667) -> ()  [unwired: 2 in, 2 out]
                n1072 = property on="Shutter TTL 4" class="Ring (strict)"("DisabledEnum"=w1667) -> ()  [unwired: 2 in, 2 out]
                n1073 = property on="Readout Rate 4" class="Ring (strict)"("DisabledEnum"=w1667) -> ()  [unwired: 2 in, 2 out]
                n1074 = property on="Vertical Shift Speed 4" class="Ring (strict)"("DisabledEnum"=w1667) -> ()  [unwired: 2 in, 2 out]
                n1075 = property on="CCD EM Mode 4" class="Ring (strict)"("DisabledEnum"=w1667) -> ()  [unwired: 2 in, 2 out]
                n1076 = property on="Trigger Mode 4" class="Ring (strict)"("DisabledEnum"=w1667) -> ()  [unwired: 2 in, 2 out]
                n1077 = property on="Read Mode 4" class="Ring (strict)"("DisabledEnum"=w1667) -> ()  [unwired: 2 in, 2 out]
                n1078 = property on="Pre-amplification Gain 4" class="Ring (strict)"("DisabledEnum"=w1667) -> ()  [unwired: 2 in, 2 out]
              }
              frame #19 {
                n1079 = case shown="True" w1829 {
                  tunnel: [w1830 w1866] -> w1827
                  tunnel: [w1830 w1850] -> w1828
                  tunnel: w1826 -> [_ w1856]
                  frame False {
                    w1830 = FALSE
                  }
                  frame True {
                    w1836 = TRUE
                    # "Pelo menos 1 canal deve \nestar habilitado"
                    n1080 = local read "Preview Temp."() -> (w1855:dbl)
                    n1081 = Unbundle By Name(w1856) -> ("ChannelA_Status.target  temp"=w1852:i16, "ChannelB_Status.target  temp"=w1854:i16, "ChannelC_Status.target  temp"=w1853:i16, "ChannelD_Status.target  temp"=w1851:i16)
                    n1082 = property on="CCD checked 3" class="Bool (strict)"() -> ("Value"=w1862:bool)  [unwired: 2 in, 2 out]
                    n1083 = local read "CH3 on"() -> (w1846:bool)
                    n1084 = local read "CH1on"() -> (w1848:bool)
                    n1085 = property on="CCD checked 2" class="Bool (strict)"() -> ("Value"=w1865:bool)  [unwired: 2 in, 2 out]
                    n1086 = local read "CH2on"() -> (w1847:bool)
                    n1087 = property on="CCD checked 1" class="Bool (strict)"() -> ("Value"=w1869:bool)  [unwired: 2 in, 2 out]
                    n1088 = property on="CCD checked 4" class="Bool (strict)"() -> ("Value"=w1859:bool)  [unwired: 2 in, 2 out]
                    n1089 = local read "CH4 on"() -> (w1845:bool)
                    n1090 = To Word Integer(number=w1855) -> (16bit integer=w1849:i16)
                    n1091 = Select(t=w1869, s=w1848, f=TRUE) -> (s? t:f=w1867:bool)
                    n1092 = local read "CH3 on"() -> (w1838:bool)
                    n1093 = local read "CH4 on"() -> (w1837:bool)
                    n1094 = Compound Arithmetic op=OR(w1848, w1847, w1846, w1845) -> (w1835:bool)
                    n1095 = local read "CH2on"() -> (w1839:bool)
                    n1096 = Select(t=w1862, s=w1846, f=TRUE) -> (s? t:f=w1860:bool)
                    n1097 = Select(t=w1865, s=w1847, f=TRUE) -> (s? t:f=w1863:bool)
                    n1098 = Select(t=w1859, s=w1845, f=TRUE) -> (s? t:f=w1857:bool)
                    n1099 = Equal?(x=w1849, y=w1854) -> (x = y?=w1843:bool)
                    n1100 = Equal?(x=w1849, y=w1853) -> (x = y?=w1842:bool)
                    n1101 = Equal?(x=w1849, y=w1851) -> (x = y?=w1841:bool)
                    n1102 = Equal?(x=w1849, y=w1852) -> (x = y?=w1844:bool)
                    n1103 = local read "CH1on"() -> (w1840:bool)
                    n1104 = Select(t=w1844, s=w1840, f=w1836) -> (s? t:f=w1834:bool)
                    n1105 = Select(t=w1842, s=w1838, f=w1836) -> (s? t:f=w1832:bool)
                    n1106 = Select(t=w1841, s=w1837, f=w1836) -> (s? t:f=w1831:bool)
                    n1107 = Select(t=w1843, s=w1839, f=w1836) -> (s? t:f=w1833:bool)
                    n1108 = Compound Arithmetic op=AND(w1867, w1863, w1860, w1857, w1835) -> (w1866:bool)
                    n1109 = Compound Arithmetic op=AND(w1835, w1834, w1833, w1832, w1831) -> (w1850:bool)
                  }
                }
                "SET Temp status" <- w1828
                "SET CCD status" <- w1827
              }
            }
            n1110 = call-dynamic "Read Obs_state.vi"("error in (no error)"=w233, "S4ACS_GUI in"=w234) -> ("error out"=w210:errorcluster, "Obs_state"=w230:u32, "S4ACS_GUI out"=w211:refnum<class "S4GUI.lvclass">)  [unwired: 7 in]
            n1111 = In Range and Coerce(upper limit=u32 226, x=w230, lower limit=u32 220 ("upper limit")) -> (In Range?=w228:bool)  [unwired: 1 out]
            n1112 = call-dynamic "Read TelFocus.lvclass.vi"("error in (no error)"=w210, "S4GUI in"=w211) -> ("error out"=w208:errorcluster, "TelFocus.lvclass"=w209:refnum<class "TelFocus.lvclass">)  [unwired: 7 in, 1 out]
            n1113 = Select(t="STOP", s=w228, f="INIT") -> (s? t:f=w227:string)
            n1114 = call-dynamic "Read focus #stepsdone.vi"("error in (no error)"=w208, "TelFocus in"=w209) -> ("focus #stepsdone"=→"steps done":u32)  [unwired: 7 in, 2 out]
            n1115 = property on="Init mode" class="Bool"(error in=w210, "Blinking"=w228, "Caption.Visible"=w228, "BoolText.Text"=w227) -> (error out=w229:errorcluster)  [unwired: 1 in, 1 out]
            n1116 = call-dynamic "Read cyclesDone.vi"("error in (no error)"=w229, "S4GUI in"=w211) -> ("error out"=w221:errorcluster, "cyclesDone"=w213:u32, "S4GUI out"=w223:refnum<class "S4GUI.lvclass">)  [unwired: 7 in]
            "#Cycles Done" <- w213
            n1117 = call-dynamic "Read cycles wprot.vi"("error in (no error)"=w221, "S4GUI in"=w223) -> ("cycles wprot"=→"Cycles Counter":u32)  [unwired: 7 in, 2 out]
            n1118 = Number To Decimal String(number=w213) -> (decimal integer string=w214:string)  [unwired: 1 in]
            n1119 = Concatenate Strings("#Cycles Done ", w214) -> (w212:string)
            n1120 = property on="#Cycles Done" class="Slide (strict)"("Caption.Text"=w212) -> ()  [unwired: 2 in, 2 out]
            n1121 = call "Read Instrument.lvclass.vi"("error in (no error)"=w221, "S4ACS_GUI in"=w223) -> ("error out"=w238:errorcluster, "Instrument.lvclass"=w236:refnum<class "Instrument.lvclass">, "S4ACS_GUI out"=w239:refnum<class "S4GUI.lvclass">)  [unwired: 7 in]
            n1122 = call-dynamic "Write mode.vi"("error in (no error)"=w238, "mode"=w224, "Instrument in"=w236) -> ("error out"=w237:errorcluster, "Instrument out"=w235:refnum<class "Instrument.lvclass">)  [unwired: 7 in]
            n1123 = call "Write Instrument.lvclass.vi"("error in (no error)"=w237, "Instrument.lvclass"=w235, "S4ACS_GUI in"=w239) -> ("error out"=w219:errorcluster, "S4ACS_GUI out"=w220:refnum<class "S4GUI.lvclass">)  [unwired: 7 in]
            n1124 = call-dynamic "Read Error Msg.vi"("error in (no error)"=w219, "S4GUI in"=w220) -> ("error out"=w216:errorcluster, "Error Msg"=w196:string, "S4GUI out"=w201:refnum<class "S4GUI.lvclass">)  [unwired: 7 in]
            "Last Error" <- w196
            n1125 = Match Pattern(string=w196, regular expression=w217) -> (match substring=w218:string)  [unwired: 1 in, 3 out]
            n1126 = Equal?(x=w218, y=w217) -> (x = y?=w195:bool)
            n1127 = Match Pattern(string=w196, regular expression=w197) -> (match substring=w198:string)  [unwired: 1 in, 3 out]
